vi "例4.9 自动索引例2.vi"() -> ()   [LabVIEW 2017]
panel:
  out "数组":dbl[][](array[numeric])
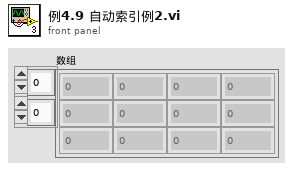
[diagram p1: front panel]
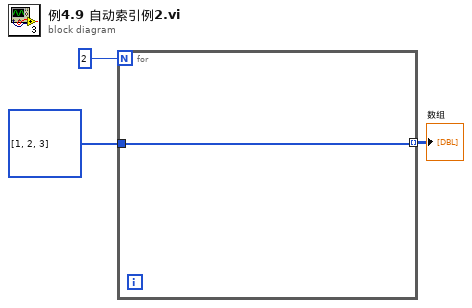
[diagram p0: block diagram]
diagram:
  n1 = for {
    N: 2 -> [_]
    tunnel: i32[] [1, 2, 3] -> [w4]
    tunnel: [w4] -> w2 mode=indexing
  }
  "数组" <- w2
